vi "Subscribe to Actor Stopped.vi"(8 "error in (no error)":errorcluster, 11 "API in":refnum<class "Interface.lvclass">) -> (0 "error out":errorcluster, 2 "Actor-Stopped Message":refnum<event-registration>, 3 "API out":refnum<class "Interface.lvclass">)   [LabVIEW 2018, in "Scripting.lvlib" / "Actor.lvlib" / "Interface.lvclass"]
uses:
  Interface.lvclass
  Actor-Stopped.ctl
  Actor.lvclass
  Interface.lvclass/Interface.ctl
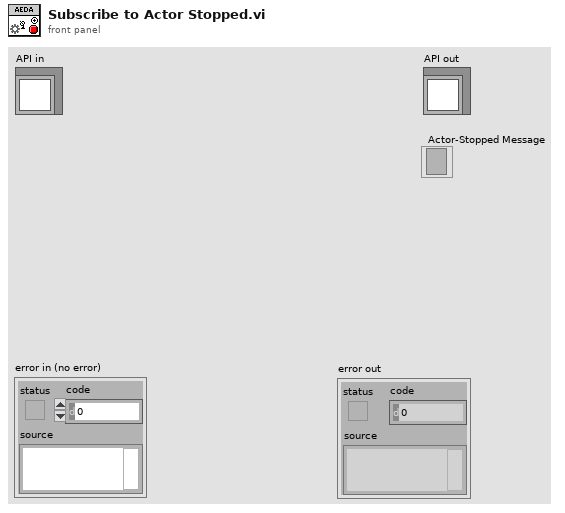
[diagram p1: front panel]
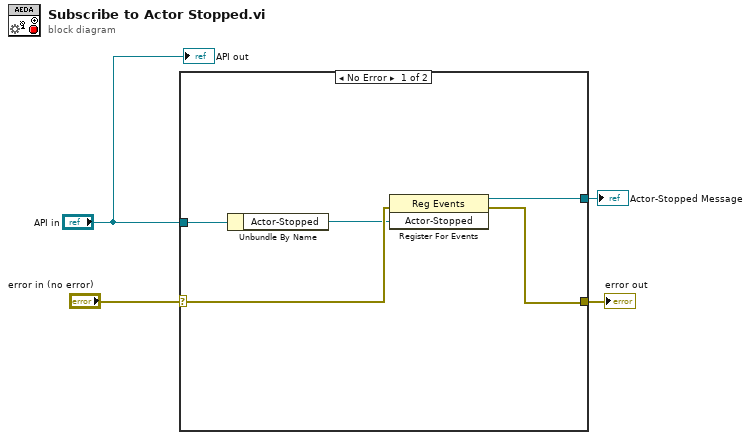
[diagram p0: block diagram]
diagram:
  n1 = case shown="No Error" "error in (no error)" {
    selector: "error in (no error)" -> [w9 w10]
    tunnel: [w8 w10] -> w3
    tunnel: "API in" -> [w7 _]
    tunnel: [w5 _] -> w1
    frame No Error {
      n2 = Unbundle By Name(w7) -> ("Actor-Stopped"=w6:refnum<user-event>)
      n3 = register-events(error in=w9, w6) -> (reference out=w5:refnum<event-registration>, error out=w8:errorcluster)  [unwired: 1 in]
    }
    frame Error {
    }
  }
  "error out" <- w3
  "Actor-Stopped Message" <- w1
  "API out" <- "API in"
